vi "proceed.vi"(8 "error in (no error)":errorcluster, 11 "ExperimentControllerDL090130Interval in":refnum<class "ExperimentControllerDL090130Interval.lvclass">) -> (0 "error out":errorcluster, 3 "ExperimentControllerDL090130Interval out":refnum<class "ExperimentControllerDL090130Interval.lvclass">)   [LabVIEW 2010, in "ExperimentControllerDL090130Interval.lvclass"]
uses:
  ExperimentControllerDL090130Interval.lvclass
  ExperimentControllerDL090130Interval.lvclass/ExperimentControllerDL090130Interval.ctl
  Sweep/GenericSweep/GenericSweep/GenericSweep.lvclass
  common/classes/ErrorController/ErrorController/class_data.vi
  common/classes/ErrorController/ErrorController/ErrorController.lvclass
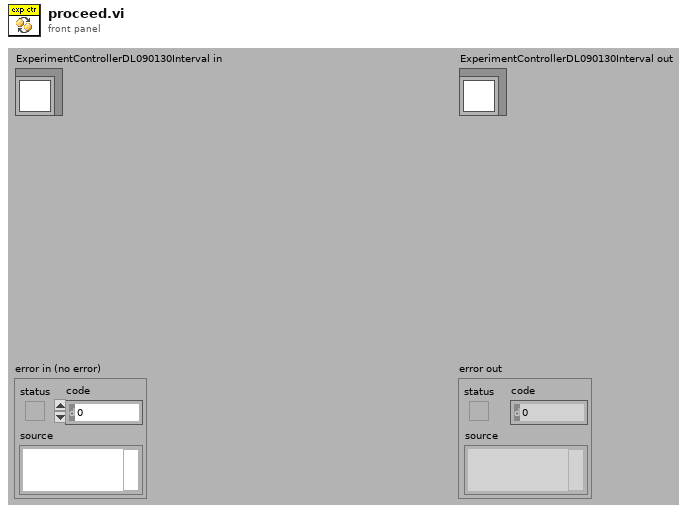
[diagram p1: front panel]
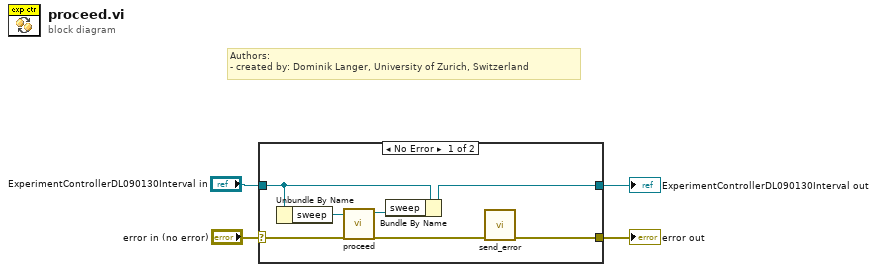
[diagram p0: block diagram]
diagram:
  # "Authors: \n- created by: Dominik Langer, University of Zurich, Switzerland"
  n1 = case shown="No Error" "error in (no error)" {
    selector: "error in (no error)" -> [w9 w13]
    tunnel: [w5 w13] -> w3
    tunnel: [w10 w12] -> w1
    tunnel: "ExperimentControllerDL090130Interval in" -> [w11 w12]
    frame No Error {
      n2 = Unbundle By Name(w11) -> ("sweep"=w8:refnum<class "GenericSweep.lvclass">)
      n3 = call-dynamic "proceed.vi"("error in (no error)"=w9, "GenericSweep in"=w8) -> ("error out"=w6:errorcluster, "GenericSweep out"=w7:refnum<class "GenericSweep.lvclass">)  [unwired: 8 in]
      n4 = Bundle By Name(cluster=w11, "sweep"=w7) -> (w10:refnum<class "ExperimentControllerDL090130Interval.lvclass">)
      n5 = call "send_error.vi"("error in (no error)"=w6) -> ("error out"=w5:errorcluster)  [unwired: 10 in]
    }
    frame Error {
    }
  }
  "error out" <- w3
  "ExperimentControllerDL090130Interval out" <- w1
